vi "Angle Calc_Individual Process R4.vi"(0 "Angle to Pixel Ratios":T2={"Horizontal Angle / Px Ratio"=0.09917687, "Vertical Angle / Px Ratio"=0.10003997}, 1 "Previous Angles":sgl[](array[numeric])=[93.87193, 100.424255, 106.972824], 5 "Num of Beacons":i8=5, 7 "Beacon Coordinates - Image":T1={"Beacon Position - X px"=[315.0, 370.0, 425.0], "Beacon Position - Y px"=[207.0, 206.0, 205.0]}, 9 "Current Servo Angle":dbl=90.0 format="%#_13g", 11 "Beacons Found (Bool Array)":bool[](array[boolean])=[TRUE, TRUE, TRUE], 12 "Previous Valid Angles":bool[](array[boolean])=[TRUE, TRUE, TRUE], 13 "Tracking Coordinates":cluster{"X":dbl, "Y":dbl}) -> (3 "Servo Goal Angle":sgl, 4 "Valid Beacons (Bool Array)\nPosition Calc":bool[](array[boolean])=[TRUE, TRUE, TRUE], 6 "Num of Valid Beacons":i8=3, 8 "Angle Of Beacons \nRelative to Robot":sgl[](array[numeric])=[93.87193, 100.424255, 106.972824])   [LabVIEW 2015]
uses:
  <vilib>/Analysis/NI_AALPro.lvlib
panel:
  in  "Max Previous\nAngle Dev.":sgl=16.0
  out "Beacon Coordinates\n - Image Centered":T1={"Beacon Position - X px"=[41.0, 107.0, 173.0], "Beacon Position - Y px"=[-51.0, -48.0, -46.0]}
  in  "Image Width":sgl=320.0 format="%#_13g"
  in  "Image Height":sgl=240.0 format="%#_13g"
  in  "Servo Middle\nAngleThreshold":dbl=4.0 format="%#_13g"
  out "Intercept":sgl=-52.386364 format="%#_13g"
  out "Angle Of Beacons \nRelative to Center (servo)":sgl[](array[numeric])=[3.8719318, 10.424257, 16.972828]
  out "Normalized Center of\nImage Angles":cluster{"X":sgl, "Y":sgl}={"X"=0.19651788, "Y"=-5.2332215} {"Y" format="%#_13g"; "X" format="%#_13g"}
  out "Beacon delta Angles":cluster{"X Angle":sgl[], "Y Angle":sgl[]}={"X Angle"=[4.0656266, 10.613175, 17.156971], "Y Angle"=[-5.0853934, -4.8352323, -4.585181]}
  out "Normalized Center of\nImage Coordinates":cluster{"X":sgl, "Y":sgl}={"X"=1.9814891, "Y"=-52.31131} {"Y" format="%#_13g"; "X" format="%#_13g"}
  out "Perpendicular Slope":sgl=-26.4 format="%#_13g"
  out "Normalized Beacon Coordinates":T3={"Beacon Position - X"=[-50.83362, -48.333008, -45.833496], "Beacon Position - Y"=[40.9937, 107.01261, 172.99368]}
  in  "DeviationThreshold":sgl=10.0 format="%#_13g"
  out "Slope":sgl=0.03787879 format="%#_13g"
  in  "Slope Threshold":sgl=10.0 format="%#_13g"
  # "CALIBRATION"
  # "INPUTS"
  # "INTERMEDIATE VARIABLE VALUES"
  # "FILTER THRESHOLDS"
  # "OUTPUT VALUES"
  # "IMPORTANT: This \nThreshold will be used\nto determine if center \nangle is within \n\"Tracking\" Range\n*update: currently not\nreally used.."
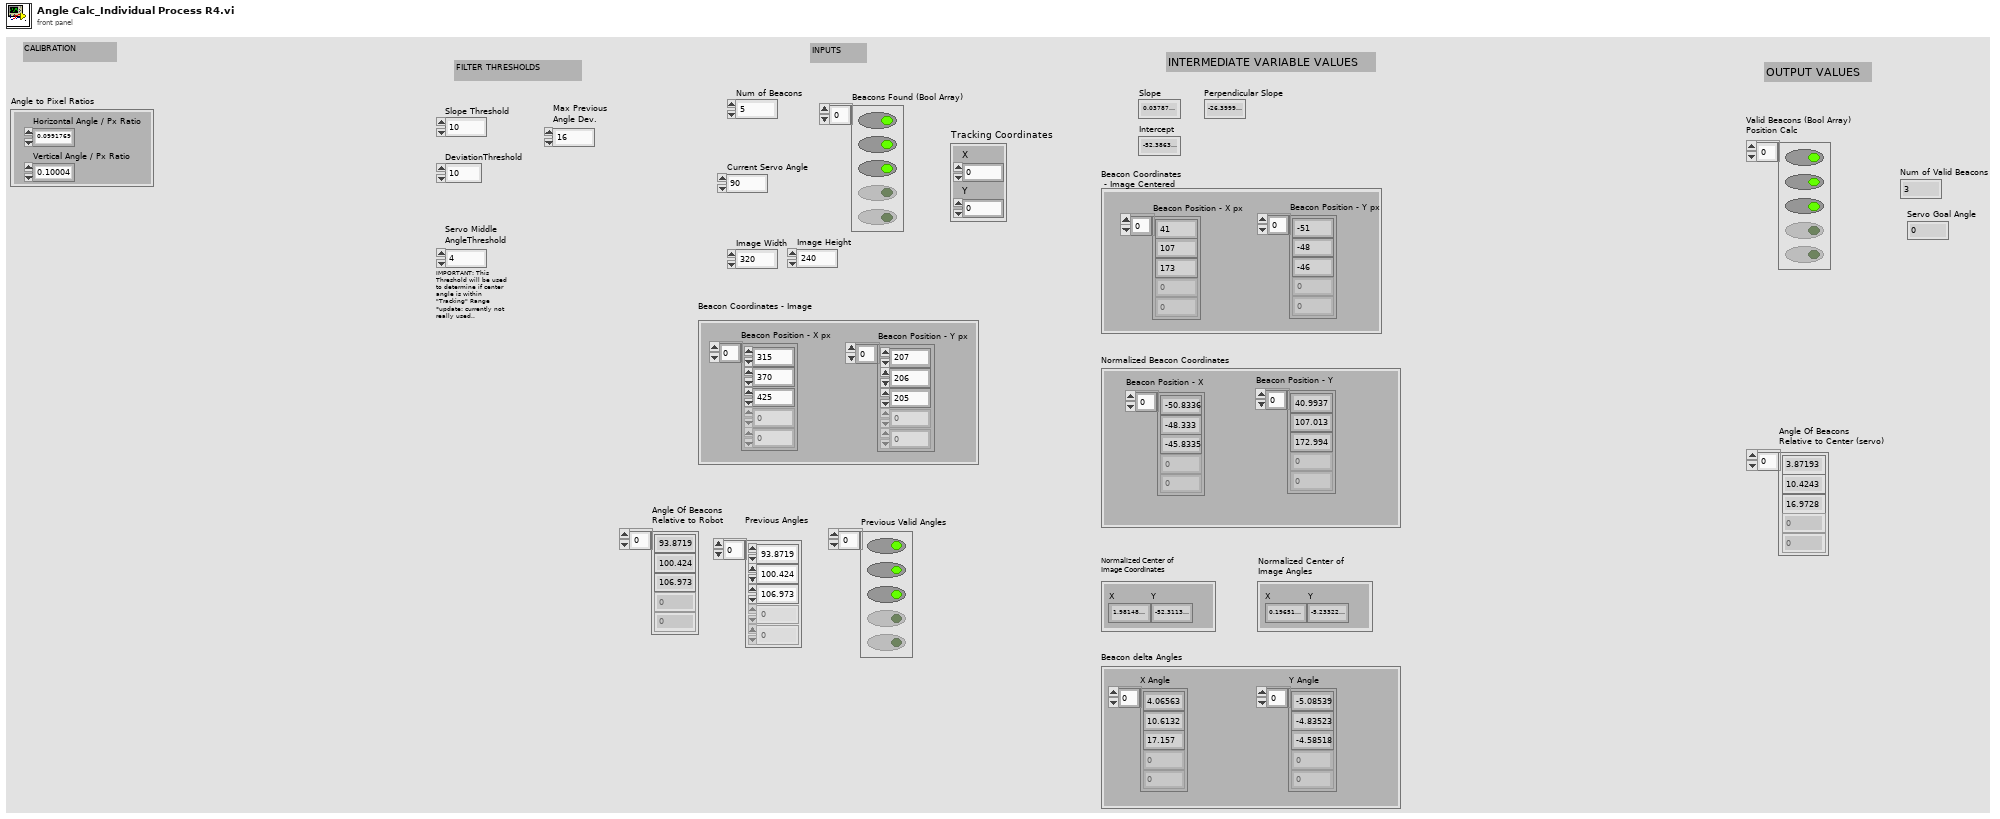
[diagram p1: front panel]
types:
  T1 = cluster{"Beacon Position - X px":sgl[], "Beacon Position - Y px":sgl[]}
  T2 = cluster{"Horizontal Angle / Px Ratio":sgl, "Vertical Angle / Px Ratio":sgl}
  T3 = cluster{"Beacon Position - X":sgl[], "Beacon Position - Y":sgl[]}
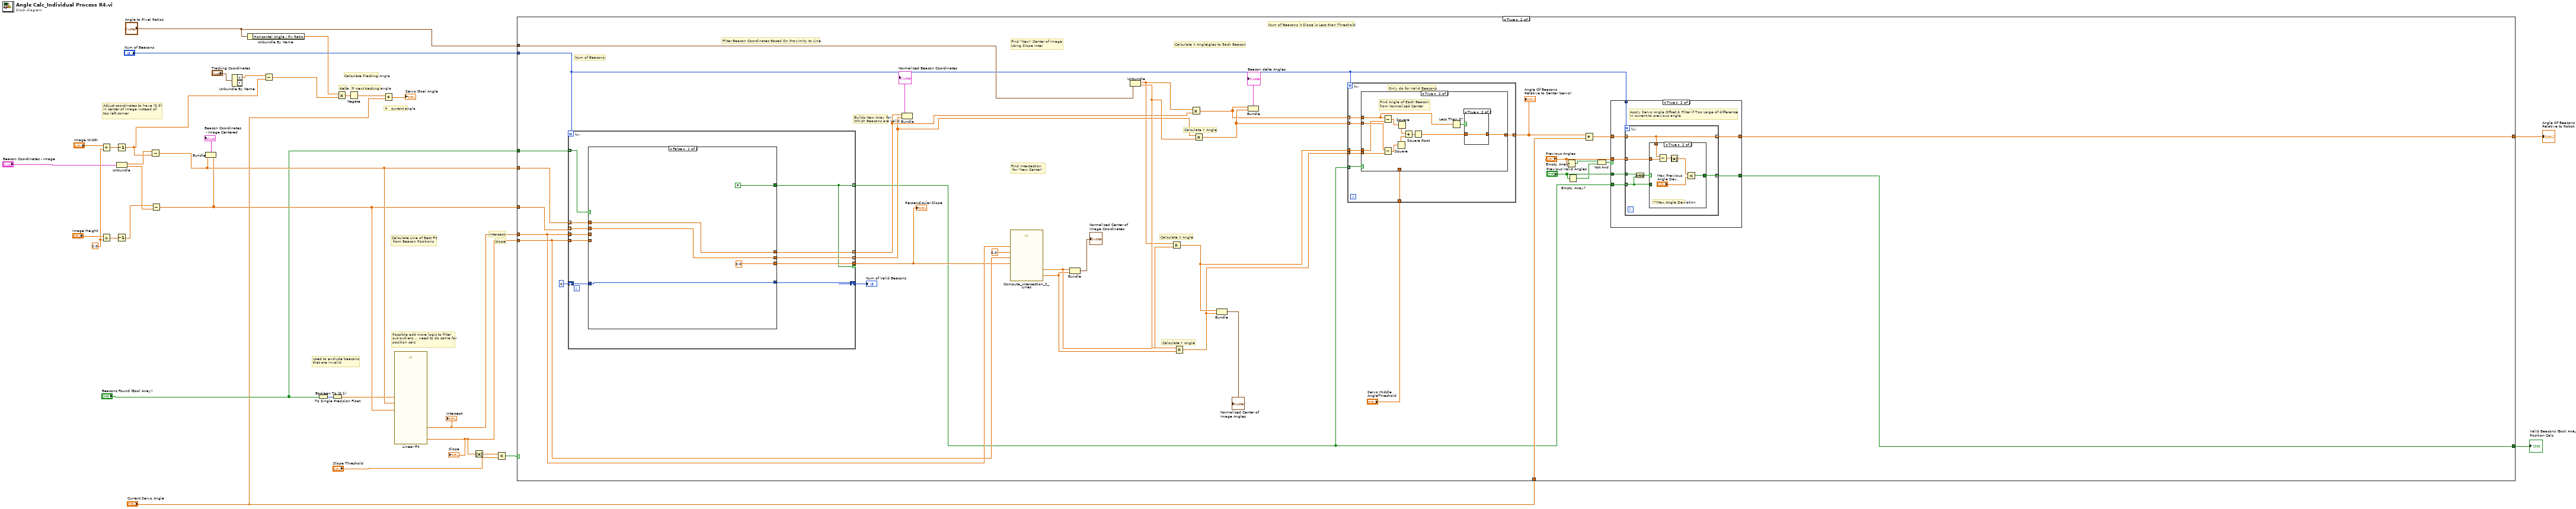
[diagram p0: block diagram]
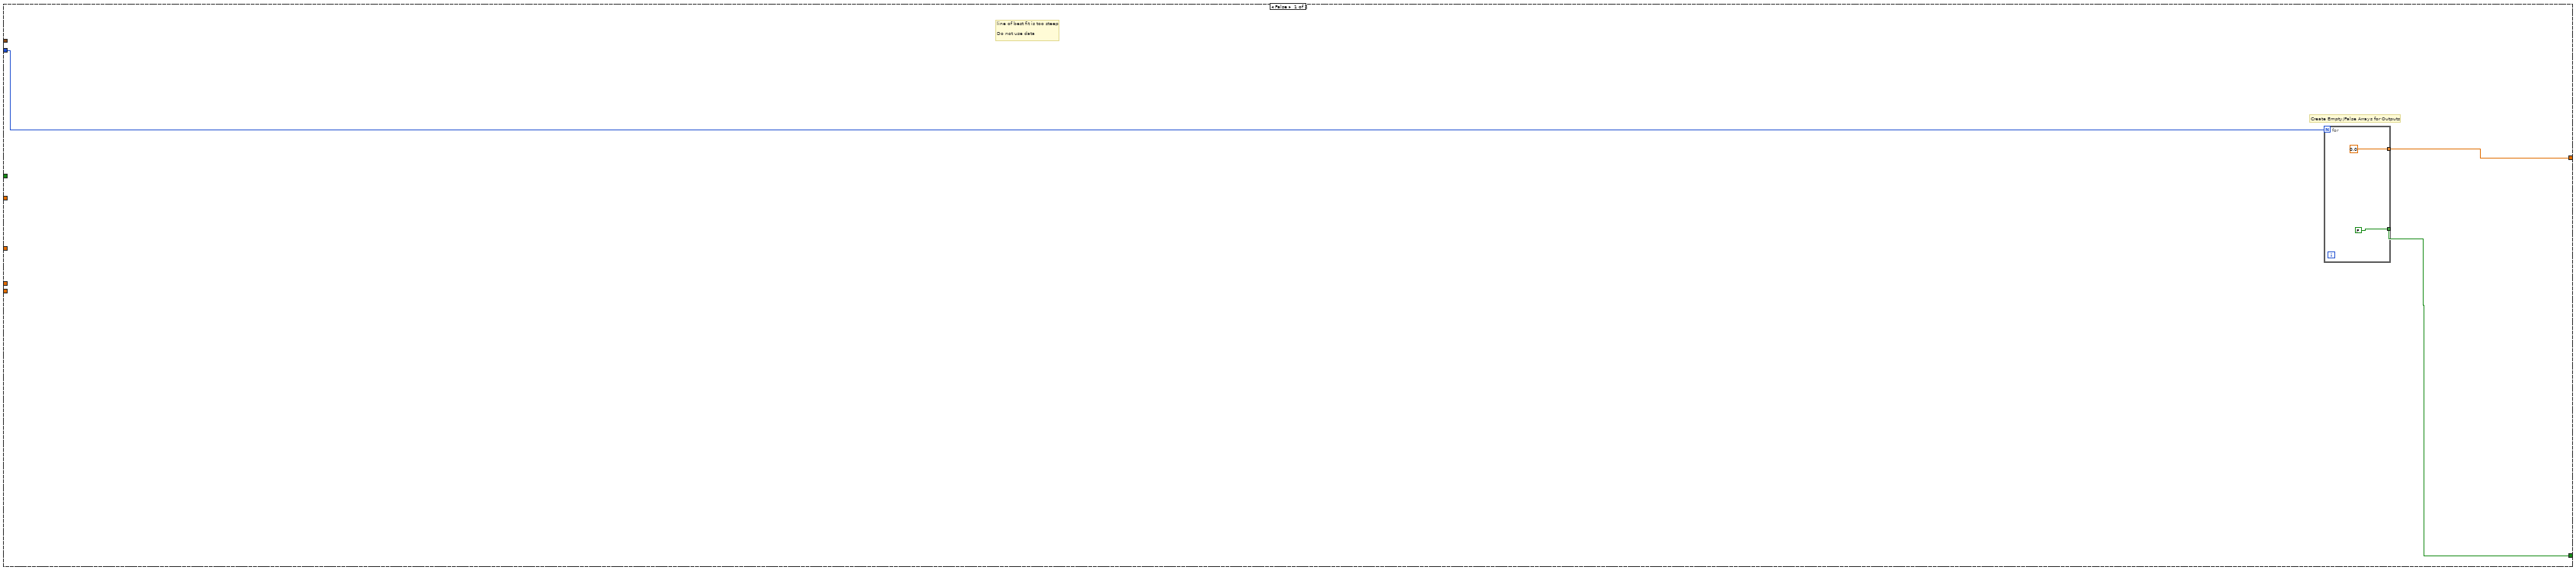
[diagram p2: hidden frame]
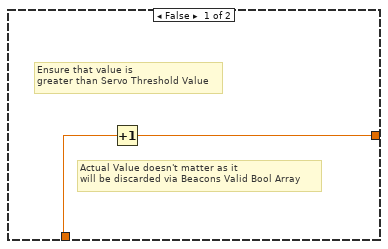
[diagram p5: hidden frame]
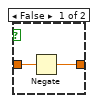
[diagram p6: hidden frame]
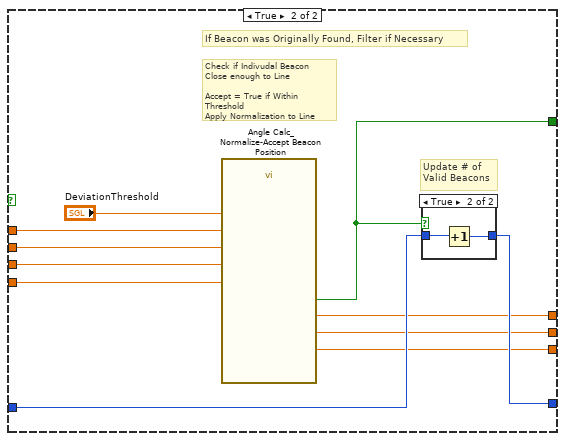
[diagram p7: hidden frame]
diagram:
  w26 = sgl 2.0
  # "= next tracking angle"
  # "+   current angle"
  # "delta"
  # "Calculate Tracking Angle"
  # "Possible add more logic to filter\nout outliers.... need to do same for\nposition calc"
  # "Calculate Line of Best Fit\n from Beacon Positions"
  # "slope"
  # "intercept"
  # "Used to exclude beacons \nthat are invalid"
  # "Adjust coordinates to have (0,0) \nin center of image instead of \ntop left corner"
  n1 = Divide(x="Image Width", y=w26) -> (x/y=w28:sgl)
  n2 = Divide(x="Image Height", y=w26) -> (x/y=w27:sgl)
  n3 = Decrement(x=w28) -> (x-1=w6:sgl)
  n4 = Decrement(x=w27) -> (x-1=w24:sgl)
  n5 = Unbundle("Beacon Coordinates - Image") -> ("Beacon Position - X px"=w31:sgl[], "Beacon Position - Y px"=w30:sgl[])
  n6 = Subtract(x=w31, y=w6) -> (x-y=w21:sgl[])
  n7 = Subtract(x=w24, y=w30) -> (x-y=w20:sgl[])
  n8 = Bundle(w21, w20) -> (→"Beacon Coordinates\n - Image Centered":cluster{sgl[], sgl[]})  [unwired: 1 in]
  n9 = Unbundle By Name("Tracking Coordinates") -> ("X"=w7:dbl)  [unwired: 1 out]
  n10 = Unbundle By Name("Angle to Pixel Ratios") -> ("Horizontal Angle / Px Ratio"=w3:sgl)
  n11 = Subtract(x=w7, y=w6) -> (x-y=w5:dbl)
  n12 = Boolean To (0,1)(Boolean="Beacons Found (Bool Array)") -> (0, 1=w16:i16[])
  n13 = To Single Precision Float(number=w16) -> (single precision float=w11:sgl[])
  n14 = Multiply(x=w3, y=w5) -> (x*y=w9:dbl)
  n15 = Negate(x=w9) -> (-x=w10:dbl)
  n16 = Add(x=w10, y="Current Servo Angle") -> (x+y=→"Servo Goal Angle":dbl)
  n17 = call <vilib>:"Linear Fit.vi"("Y"=w20, "X"=w21, "Weight"=w11) -> ("slope"=w13:dbl, "intercept"=w14:dbl)  [unwired: 8 in, 3 out]
  "Slope" <- w13
  "Intercept" <- w14
  n18 = Absolute Value(x=w13) -> (abs(x)=w12:dbl)
  n19 = Less?(x=w12, y="Slope Threshold") -> (x < y?=w15:bool)
  n20 = case shown="True" w15 {
    tunnel: w13 -> [_ w73]
    tunnel: w14 -> [_ w72]
    tunnel: w21 -> [_ w75]
    tunnel: w20 -> [_ w74]
    tunnel: "Angle to Pixel Ratios" -> [_ w71]
    tunnel: "Num of Beacons" -> [w36 w60]
    tunnel: [w34 w50] -> w33
    tunnel: [w35 w59] -> w32
    tunnel: "Beacons Found (Bool Array)" -> [_ w61]
    tunnel: "Current Servo Angle" -> [_ w42]
    frame False {
      # "Create Empty/False Arrays for Outputs"
      # "line of best fit is too steep\n\nDo not use data"
      n21 = for {
        N: w36 -> [_]
        tunnel: [FALSE] -> w35 mode=indexing
        tunnel: [sgl 0.0] -> w34 mode=indexing
      }
    }
    frame True {
      # "Calculate X Angle"
      # "Num of Beacons"
      # "Find dX and dY Angles to Each Beacon"
      # "Calculate Y Angle"
      # "Calculate X Angle"
      # "Calculate Y Angle"
      # "Calculate X Angle"
      # "Find Intersection\n for \"New Center\""
      # "Find \"New\" Center of Image\nUsing Slope Inter"
      # "Num of Beacons"
      # "Builds New Array for\nWhich Beacons are Valid"
      # "Filter Beacon Coordinates Based On Proximity to Line"
      # "If Line of Bestst Fit Slope is Less than Threshold"
      n22 = for {
        N: w60 -> [_]
        shift-right: [w127] -> w64
        shift-left: 0 -> [w132]
        tunnel: w72 -> [w131]
        tunnel: w73 -> [w130]
        tunnel: w75 -> [w129] mode=indexing
        tunnel: w74 -> [w128] mode=indexing
        tunnel: [w122] -> w40 mode=indexing
        tunnel: [w126] -> w56 mode=indexing
        tunnel: [w125] -> w55 mode=indexing
        tunnel: w61 -> [w124] mode=indexing
        tunnel: [w123] -> w41 if=w122
        n23 = case shown="False" w124 {
          tunnel: w132 -> [w133 w142]
          tunnel: w131 -> [_ w147]
          tunnel: w130 -> [_ w146]
          tunnel: w129 -> [w135 w145]
          tunnel: w128 -> [w136 w144]
          tunnel: [FALSE w143] -> w122
          tunnel: [w133 w141] -> w127
          tunnel: [w135 w140] -> w126
          tunnel: [w136 w139] -> w125
          tunnel: [sgl 0.0 w138] -> w123
          frame False {
          }
          frame True {
            # "Update # of \nValid Beacons"
            # "Check if Indivudal Beacon\nClose enough to Line\n\nAccept = True if Within Threshold\nApply Normalization to Line"
            # "If Beacon was Originally Found, Filter if Necessary"
            n24 = call "Angle Calc_Normalize-Accept Beacon Position.vi"("slope"=w146, "Xin"=w145, "Deviation Threshold"="DeviationThreshold", "intercept"=w147, "Yin"=w144) -> ("Accept Beacon"=w143:bool, "Xout"=w140:sgl, "Perpendicular Slope"=w138:sgl, "Yout"=w139:sgl)  [unwired: 6 in, 1 out]
            n25 = case shown="True" w143 {
              tunnel: [w149 w150] -> w141
              tunnel: w142 -> [w149 w151]
              frame False {
              }
              frame True {
                n26 = Increment(x=w151) -> (x+1=w150:i32)
              }
            }
          }
        }
      }
      "Num of Valid Beacons" <- w64
      "Perpendicular Slope" <- w41
      n27 = Bundle(w56, w55) -> (→"Normalized Beacon Coordinates":cluster{sgl[], sgl[]})  [unwired: 1 in]
      n28 = call "Compute_Intersection_2_Lines.vi"("m'"=w41, "b'"=0.0, "b"=w72, "m"=w73) -> ("Yint"=w57:sgl, "Xint"=w58:sgl)  [unwired: 6 in]
      n29 = Bundle("Xint"=w58, "Yint"=w57) -> (→"Normalized Center of\nImage Coordinates":cluster{"Xint":sgl, "Yint":sgl})  [unwired: 1 in]
      n30 = Unbundle(w71) -> ("Horizontal Angle / Px Ratio"=w39:sgl, "Vertical Angle / Px Ratio"=w62:sgl)
      n31 = Multiply(x=w39, y=w58) -> (x*y=w51:sgl)
      n32 = Multiply(x=w62, y=w57) -> (x*y=w52:sgl)
      n33 = Multiply(x=w39, y=w56) -> (x*y=w53:sgl[])
      n34 = Multiply(x=w55, y=w62) -> (x*y=w54:sgl[])
      n35 = Bundle(w51, w52) -> (→"Normalized Center of\nImage Angles":cluster{sgl, sgl})  [unwired: 1 in]
      n36 = Bundle(w53, w54) -> (→"Beacon delta Angles":cluster{sgl[], sgl[]})  [unwired: 1 in]
      n37 = for {
        N: w60 -> [_]
        tunnel: w53 -> [w104] mode=indexing
        tunnel: w54 -> [w103] mode=indexing
        tunnel: w51 -> [w102]
        tunnel: w52 -> [w101]
        tunnel: [w100] -> w43 mode=indexing
        tunnel: w40 -> [w99] mode=indexing
        tunnel: "Servo Middle\nAngleThreshold" -> [w98]
        # "Only do for Valid Beacons"
        n38 = case shown="True" w99 {
          tunnel: w104 -> [_ w109]
          tunnel: w103 -> [_ w113]
          tunnel: w102 -> [_ w112]
          tunnel: w101 -> [_ w111]
          tunnel: [w106 w107] -> w100
          tunnel: w98 -> [w105 _]
          frame False {
            # "Actual Value doesn't matter as it\nwill be discarded via Beacons Valid Bool Array"
            # "Ensure that value is \ngreater than Servo Threshold Value"
            n39 = Increment(x=w105) -> (x+1=w106:dbl)
          }
          frame True {
            # "Find Angle of Each Beacon \nfrom Normalized Center"
            n40 = Subtract(x=w109, y=w112) -> (x-y=w115:sgl)
            n41 = Subtract(x=w113, y=w111) -> (x-y=w114:sgl)
            n42 = Square(x=w114) -> (x^2=w117:sgl)
            n43 = Square(x=w115) -> (x^2=w118:sgl)
            n44 = Add(x=w118, y=w117) -> (x+y=w116:sgl)
            n45 = Square Root(x=w116) -> (sqrt(x)=w108:sgl)
            n46 = Less Than 0?(x=w109) -> (x < 0?=w110:bool)
            n47 = case shown="True" w110 {
              tunnel: w108 -> [w119 w121]
              tunnel: [w120 w121] -> w107
              frame False {
                n48 = Negate(x=w119) -> (-x=w120:sgl)
              }
              frame True {
              }
            }
          }
        }
      }
      "Angle Of Beacons \nRelative to Center (servo)" <- w43
      n49 = Empty Array?(array="Previous Angles") -> (empty?=w46:bool)
      n50 = Empty Array?(array="Previous Valid Angles") -> (empty?=w45:bool)
      n51 = Add(x=w43, y=w42) -> (x+y=w44:dbl[])
      n52 = Not And(1:w45, 2:w46) -> (0:w47:bool)
      n53 = case shown="True" w47 {
        tunnel: w60 -> [_ w84]
        tunnel: "Previous Angles" -> [_ w83]
        tunnel: "Previous Valid Angles" -> [_ w82]
        tunnel: w40 -> [w77 w81]
        tunnel: [w77 w80] -> w59
        tunnel: [w76 w79] -> w50
        tunnel: w44 -> [w76 w78]
        frame False {
        }
        frame True {
          # "Apply Servo Angle Offset & Filter if Too Large of difference\nin current to previous angle"
          n54 = for {
            N: w84 -> [_]
            tunnel: [w85] -> w79 mode=indexing
            tunnel: w83 -> [w90] mode=indexing
            tunnel: w82 -> [w87] mode=indexing
            tunnel: [w89] -> w80 mode=indexing
            tunnel: w81 -> [w86] mode=indexing
            tunnel: w78 -> [w85] mode=indexing
            n55 = And(x=w87, y=w86) -> (x .and. y?=w88:bool)
            n56 = case shown="True" w88 {
              tunnel: w90 -> [_ w97]
              tunnel: [w91 w93] -> w89
              tunnel: w85 -> [_ w94]
              tunnel: w86 -> [w91 _]
              frame False {
              }
              frame True {
                # "**Max Angle Deviation"
                n57 = Subtract(x=w94, y=w97) -> (x-y=w96:dbl)
                n58 = Absolute Value(x=w96) -> (abs(x)=w95:dbl)
                n59 = Less?(x=w95, y="Max Previous\nAngle Dev.") -> (x < y?=w93:bool)
              }
            }
          }
        }
      }
    }
  }
  "Angle Of Beacons \nRelative to Robot" <- w33
  "Valid Beacons (Bool Array)\nPosition Calc" <- w32
